vi "odczyt listy zdjec.vi"(5 "error in (no error)":errorcluster) -> (0 "error out":errorcluster, 1 "Nr zdjecia":i32[](array[numeric]), 2 "fps":i32[](array[numeric]), 3 "lista zdjec":string[](array[string]), 4 "sciezka do zdjec":path caption="selected path", 6 "godzina ze zdjecia":string[](array[string]))   [LabVIEW 2009]
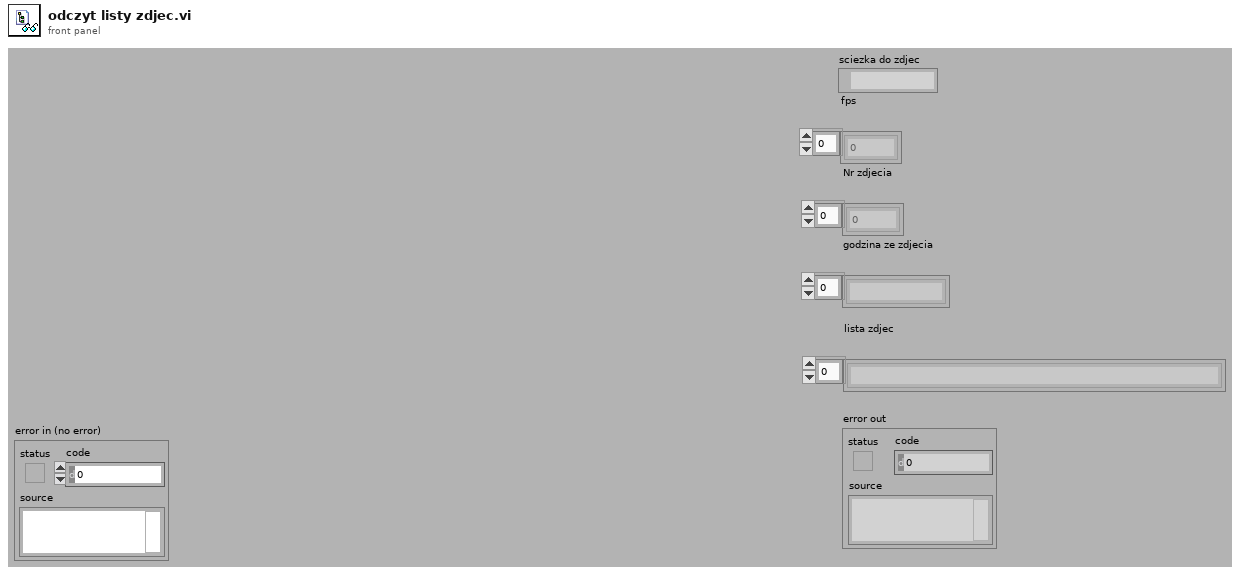
[diagram p1: front panel]
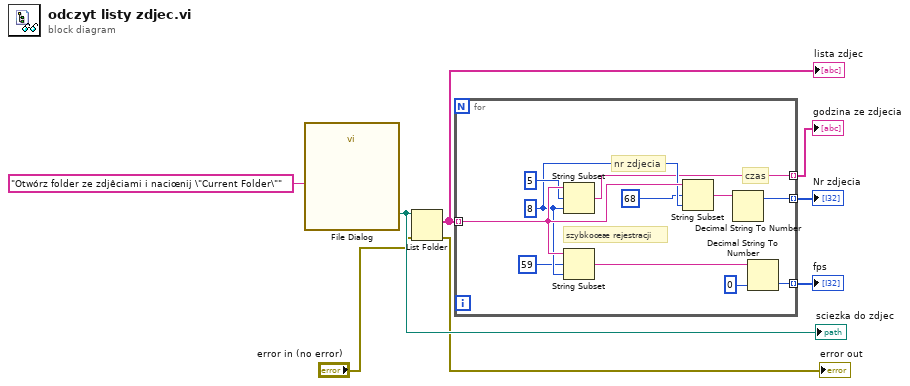
[diagram p0: block diagram]
diagram:
  n1 = call "File Dialog"("prompt"="Otwórz folder ze zdjêciami i naciœnij \"Current Folder\"") -> ("selected path"=w8:path)  [unwired: 11 in, 3 out]
  "sciezka do zdjec" <- w8
  n2 = List Folder(path=w8, error in="error in (no error)") -> (filenames=w6:string[], error out=→"error out":errorcluster)  [unwired: 2 in, 2 out]
  "lista zdjec" <- w6
  n3 = for {
    tunnel: w6 -> [w19] mode=indexing
    tunnel: [w9] -> w5 mode=indexing
    tunnel: [w11] -> w4 mode=indexing
    tunnel: [w12] -> w3 mode=indexing
    w17 = 8 ("length (rest)")
    # "nr zdjecia"
    # "szybkoœæ rejestracji"
    # "czas"
    n4 = String Subset(string=w19, offset (0)=5, length (rest)=w17) -> (substring=w12:string)
    n5 = String Subset(string=w19, offset (0)=59, length (rest)=w17) -> (substring=w13:string)
    n6 = String Subset(string=w19, offset (0)=68, length (rest)=w17) -> (substring=w14:string)
    n7 = Decimal String To Number(string=w14) -> (offset past number=w9:i32)  [unwired: 2 in, 1 out]
    n8 = Decimal String To Number(string=w13, default (0L)=0 ("default (0 DBL)")) -> (number=w11:i32)  [unwired: 1 in, 1 out]
  }
  "godzina ze zdjecia" <- w3
  "fps" <- w4
  "Nr zdjecia" <- w5
